vi "RT Toggle User LED.vi"() -> ()   [LabVIEW 2011]
uses:
  <vilib>/FPGAPlugInAG/sbRIO-9636/niLvFpga_Open_sbRIO-9636.vi
  <vilib>/rvi/interface/common/dynamic/niFpgaDynamicAddResources.vi
  <vilib>/Utility/error.llb/Error Cluster From Error Code.vi
  <vilib>/rvi/errors/niLvFpgaAdjustHostInterfaceError.vi
  <vilib>/FPGAPlugInAG/Dynamic/niLvFpga_Close_Dynamic.vi
  <vilib>/rvi/interface/nirviOpenFPGA/nirviOpenFPGA.xnode
  FPGA Bitfiles/blinky_9636.lvbitx
  FPGA Toggle FPGA LED.vi
  <vilib>/rvi/interface/nirviReadWriteControl/nirviReadWriteControl.xnode
  <vilib>/rvi/interface/nirviCloseFPGA/nirviCloseFPGA.xnode
  <vilib>/NI_Real-Time Target Support.lvlib
  NiFpgaLv.dll
  <vilib>/rvi/interface/Simulation/niFpgaSimulationCallBeginRW.vi
panel:
  in  "RT LED period (ms)":u32=1000
  in  "stop RT LED loop":bool
  out "FPGA LED State":bool
  in  "FPGA LED period (ms)":u32=500
  in  "stop FPGA\ncommunication loop":bool
  out "User LED State":bool
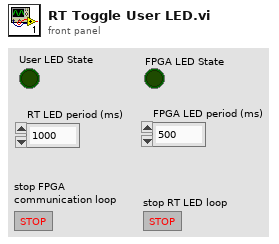
[diagram p1: front panel]
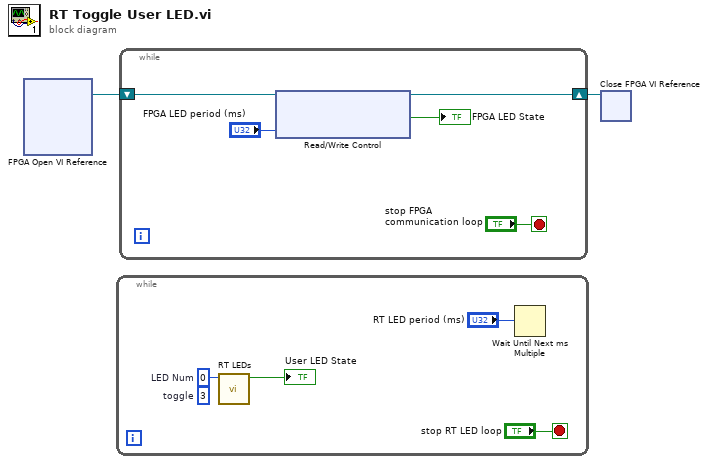
[diagram p0: block diagram]
diagram:
  n1 = xnode ("FPGA Open VI Reference")() -> ("FPGA VI Reference Out"=w2:refnum<k20>)  [unwired: 2 in, 1 out]
  n2 = while {
    stop <- "stop RT LED loop" stop-if-true
    (unwired) 3  # toggle
    w5 = 0  # LED Num
    n3 = call <vilib>:"RT LEDs.vi"("LED Num"=w5) -> ("Led State"=→"User LED State":bool)  [unwired: 5 in, 1 out]
    n4 = Wait Until Next ms Multiple(millisecond multiple="RT LED period (ms)") -> ()  [unwired: 1 out]
  }
  n5 = while {
    shift-right: [w7] -> w1
    shift-left: w2 -> [w10]
    stop <- "stop FPGA\ncommunication loop" stop-if-true
    n6 = xnode "Read/Write Control"("FPGA VI Reference In"=w10, "FPGA LED period (ms)"="FPGA LED period (ms)") -> ("FPGA VI Reference Out"=w7:refnum<k20>, "FPGA LED"=→"FPGA LED State":bool)  [unwired: 1 in, 1 out]
  }
  n7 = xnode "Close FPGA VI Reference"("FPGA VI Reference In"=w1) -> ()  [unwired: 1 in, 1 out]
